vi "ReadAllFile.vi"(5 "文件名输入":string) -> (0 "远场图":T1, 1 "近场图":T1, 2 "时间波形Data":waveform(dbl) caption="波形", 3 "光谱波形":cluster{"数组":dbl[], "数组":dbl[]}, 4 "基本数据Data":string[](array[string]))   [LabVIEW 2018]
uses:
  <vilib>/vision/Image Controls.llb/IMAQ Image.ctl
  HistoryFile.vi
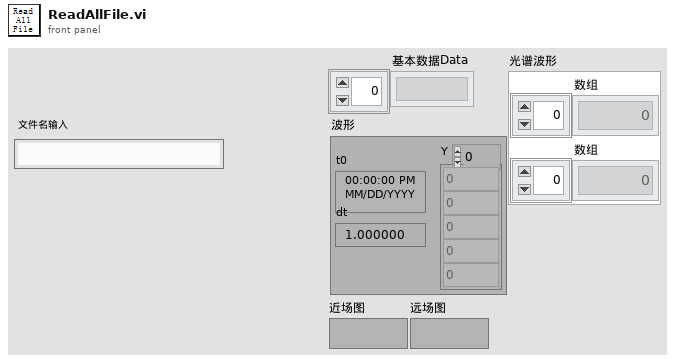
[diagram p1: front panel]
types:
  T1 = typedef "IMAQ Image.ctl" = refnum<image>
  T2 = cluster{"近场图":T1, " 远场图":T1, "发散角X":string, "发散角Y":string}
  T3 = cluster{"能量计结果":string, "功率计结果":string, "能量计单位":string, " 功率计单位":string}
  T4 = cluster{"中心波长":string, " 谱宽":string, " 中心波长Uint":string, " 谱宽 Uint":string, "波形":cluster{"数组":dbl[], "数组":dbl[]}}
  T5 = cluster{"波形":waveform(dbl), "脉宽":string, "重频":string, "脉冲宽度Uint":string, "重复频率Uint":string}
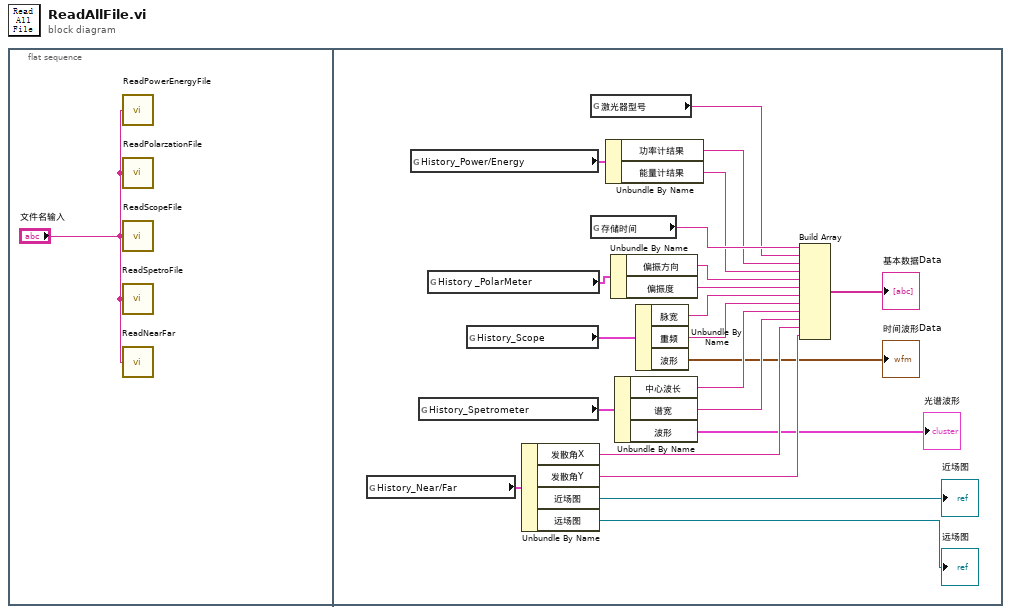
[diagram p0: block diagram]
diagram:
  n1 = flat-sequence {
    frame #0 {
      n2 = call "ReadPowerEnergyFile.vi"("本次文件名"="文件名输入") -> ()  [unwired: 1 in]
      n3 = call "ReadPolarzationFile.vi"("本次文件名"="文件名输入") -> ()  [unwired: 1 in]
      n4 = call "ReadScopeFile.vi"("本次文件名"="文件名输入") -> ()  [unwired: 1 in]
      n5 = call "ReadSpetroFile.vi"("本次文件名"="文件名输入") -> ()  [unwired: 1 in]
      n6 = call "ReadNearFar.vi"("本次文件名"="文件名输入") -> ()  [unwired: 1 in]
    }
    frame #1 {
      n7 = global read "HistoryFile.vi" "History_Near/Far"() -> (w19:T2)
      n8 = global read "HistoryFile.vi" "History_Power/Energy"() -> (w23:T3)
      n9 = global read "HistoryFile.vi" "History_Spetrometer"() -> (w20:T4)
      n10 = global read "HistoryFile.vi" "History _PolarMeter"() -> (w22:cluster{" 偏振方向":string, "偏振度":string})
      n11 = global read "HistoryFile.vi" "History_Scope"() -> (w21:T5)
      n12 = Unbundle By Name(w19) -> ("发散角X"=w8:string, "发散角Y"=w7:string, "近场图"=→"近场图":T1, "远场图"=→"远场图":T1)
      n13 = global read "HistoryFile.vi" "激光器型号"() -> (w17:string)
      n14 = global read "HistoryFile.vi" "存储时间"() -> (w18:string)
      n15 = Unbundle By Name(w23) -> ("功率计结果"=w16:string, "能量计结果"=w15:string)
      n16 = Unbundle By Name(w22) -> ("偏振方向"=w14:string, "偏振度"=w13:string)
      n17 = Unbundle By Name(w20) -> ("中心波长"=w10:string, "谱宽"=w9:string, "波形"=→"光谱波形":cluster{"数组":dbl[], "数组":dbl[]})
      n18 = Unbundle By Name(w21) -> ("脉宽"=w12:string, "重频"=w11:string, "波形"=→"时间波形Data":waveform(dbl))
      n19 = Build Array(w18, w17, w16, w15, w14, w13, w12, w11, w10, w9, w8, w7) -> (→"基本数据Data":string[])
    }
  }
